vi "Parse File from Disk.vi"(9 "Numeric":i32, 10 "filenames":string[](array[string]), 11 "path in":path) -> (3 "Tree Items Array":T1(array[cluster]))   [LabVIEW 2020, in "LV Project Items Parser.lvlib"]
doc: "Parse the elements of a folder on disk, define its extension as the type attribute for an item and then formats it to a tree control data structure."
uses:
  LV Project Items Parser.lvlib
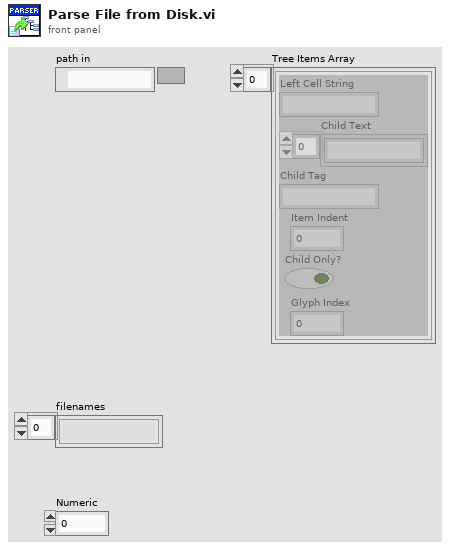
[diagram p1: front panel]
types:
  T1 = cluster{"Left Cell String":string, "Child Text":string[], "Child Tag":string, "Item Indent":i32, "Child Only?":bool, "Glyph Index":i32}[]
  T2 = cluster{"Left Cell String":string, "Child Text":string[], "Child Tag":string, "Item Indent":i32, "Child Only?":bool, "Glyph Index":i32}
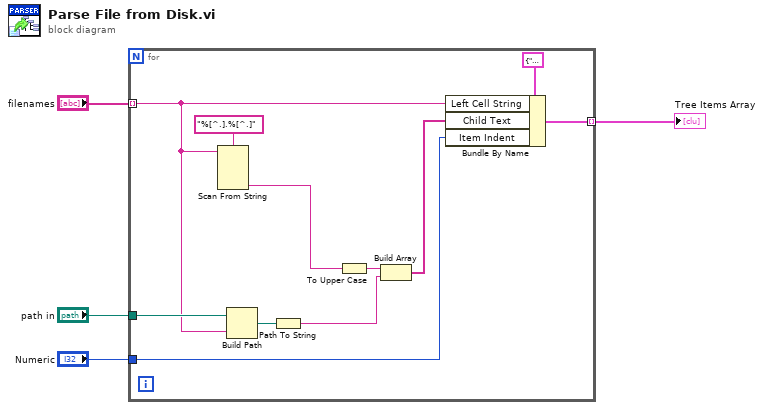
[diagram p0: block diagram]
diagram:
  n1 = for {
    tunnel: "filenames" -> [w5] mode=indexing
    tunnel: "Numeric" -> [w11]
    tunnel: [w10] -> w1 mode=indexing
    tunnel: "path in" -> [w8]
    n2 = Scan From String(format string="%[^.].%[^.]", input string=w5) -> (output 2=w13:string)  [unwired: 5 in, 3 out]
    n3 = Build Path(base path=w8, name or relative path=w5) -> (appended path=w9:path)
    n4 = Path To String(path=w9) -> (string=w6:string)
    n5 = To Upper Case(1:w13) -> (0:w7:string)
    n6 = Build Array(w7, w6) -> (w12:string[])
    n7 = Bundle By Name(cluster=T2 {"Left Cell String"="", "Child Text"=[], "Child Tag"="", "Item Indent"=0, "Child Only?"=FALSE, "Glyph Index"=0} ("Item"), "Left Cell String"=w5, "Child Text"=w12, "Item Indent"=w11) -> (w10:T2)
  }
  "Tree Items Array" <- w1
